vi "Stop ODE.vi"() -> ()   [LabVIEW 2014]
panel:
  in  "Stop ODE":bool
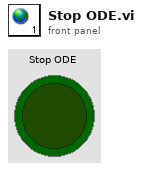
[diagram p1: front panel]
diagram:
